vi "Teleop Intake Control.vi"(9 "D-Pad":T1, 10 "Button Cluster":T2, 11 "Axes":T3) -> ()   [LabVIEW 2017]
uses:
  Common Code/Gamepads/Axes Cluster.ctl
  Common Code/Gamepads/Button Cluster.ctl
  Common Code/Gamepads/D-Pad.ctl
  Common Code/Intake States.ctl
  Common Code/Intake Mode.ctl
  Common Code/Utilities/Change Detect.vi
  Robot Global Data.vi
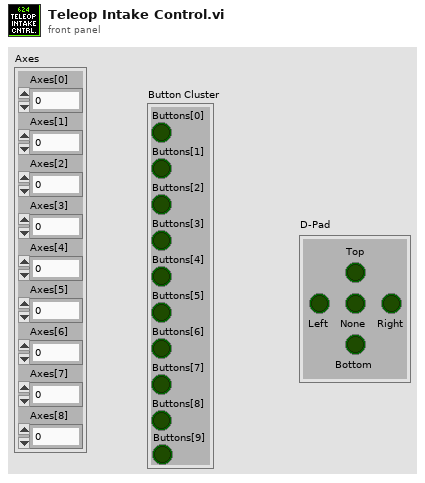
[diagram p1: front panel]
types:
  T1 = typedef "D-Pad.ctl" = cluster{"Top":bool, "Bottom":bool, "None":bool, "Right":bool, "Left":bool}
  T2 = typedef "Button Cluster.ctl" = cluster{"Buttons[0]":bool, "Buttons[1]":bool, "Buttons[2]":bool, "Buttons[3]":bool, "Buttons[4]":bool, "Buttons[5]":bool, "Buttons[6]":bool, "Buttons[7]":bool, "Buttons[8]":bool, "Buttons[9]":bool}
  T3 = typedef "Axes Cluster.ctl" = cluster{"Axes[0]":dbl, "Axes[1]":dbl, "Axes[2]":dbl, "Axes[3]":dbl, "Axes[4]":dbl, "Axes[5]":dbl, "Axes[6]":dbl, "Axes[7]":dbl, "Axes[8]":dbl}
  T4 = typedef "Intake States.ctl" = enum16{"Zero", "Override Angle", "Idle", "Drop Mid", "Drop Low", "Outtake", "Intake"}
  T5 = typedef "Intake Mode.ctl" = enum16{"Auto", "Semi Auto", "Manual"}
  T6 = typedef "Intake Command Cluster.ctl" = cluster{"Intake Mode":T5, "Intake States":T4, "Manual Roller Power":dbl, "Manual Close?":bool, "Manual Lift Power":dbl, "Override Lift?":bool, "Override Angle":dbl}
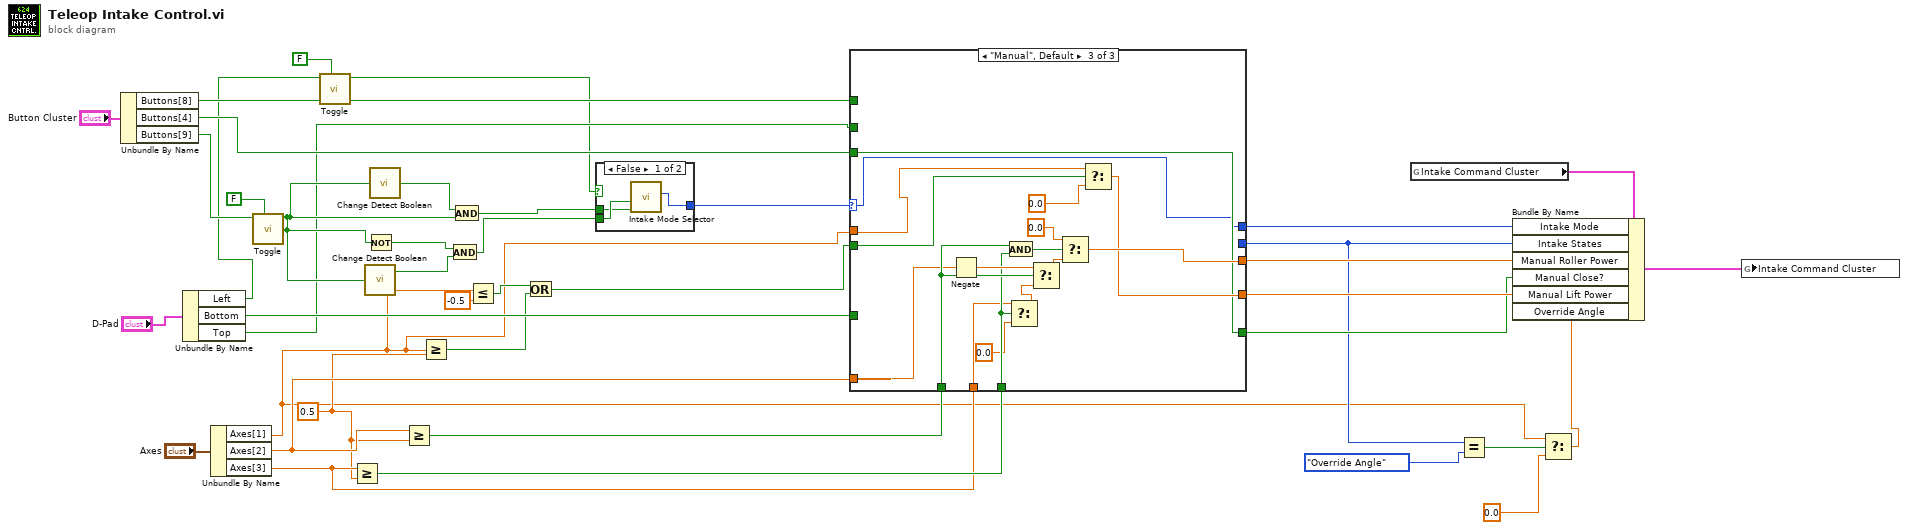
[diagram p0: block diagram]
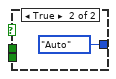
[diagram p2: hidden frame]
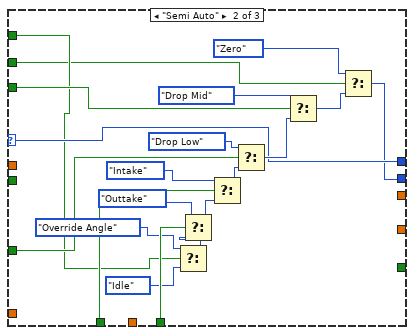
[diagram p4: hidden frame]
diagram:
  w22 = 0.5
  n1 = Unbundle By Name("Button Cluster") -> ("Buttons[8]"=w21:bool, "Buttons[4]"=w28:bool, "Buttons[9]"=w35:bool)
  n2 = Unbundle By Name("D-Pad") -> ("Left"=w1:bool, "Bottom"=w27:bool, "Top"=w7:bool)
  n3 = Unbundle By Name("Axes") -> ("Axes[1]"=w10:dbl, "Axes[2]"=w24:dbl, "Axes[3]"=w23:dbl)
  n4 = call "Toggle.vi"("Initial Value"=FALSE, "In"=w35) -> ("Toggled"=w30:bool)  [unwired: 9 in]
  n5 = call "Toggle.vi"("Initial Value"=FALSE, "In"=w1) -> ("Toggled"=w2:bool)  [unwired: 9 in]
  n6 = Greater Or Equal?(x=w23, y=w22) -> (x >= y?=w25:bool)
  n7 = call "Change Detect Boolean.vi"("In"=w30) -> ("Changed?"=w32:bool)
  n8 = Not(x=w30) -> (.not. x?=w31:bool)
  n9 = call "Change Detect Boolean.vi"("In"=w30) -> ("Changed?"=w33:bool)
  n10 = Greater Or Equal?(x=w24, y=w22) -> (x >= y?=w26:bool)
  n11 = Greater Or Equal?(x=w10, y=w22) -> (x >= y?=w19:bool)
  n12 = And(x=w31, y=w32) -> (x .and. y?=w6:bool)
  n13 = And(x=w33, y=w30) -> (x .and. y?=w5:bool)
  n14 = Less Or Equal?(x=w10, y=-0.5) -> (x <= y?=w18:bool)
  n15 = Or(x=w18, y=w19) -> (x .or. y?=w16:bool)
  n16 = case shown="False" w2 {
    tunnel: w6 -> [w43 _]
    tunnel: w5 -> [w42 _]
    tunnel: [w41 Intake_Mode."Auto" ("Intake Mode")] -> w4
    frame False {
      n17 = call "Intake Mode Selector.vi"("Semi Auto?"=w42, "Manual?"=w43) -> ("Intake Mode"=w41:T5)  [unwired: 9 in]
    }
    frame True {
    }
  }
  n18 = case shown="\"Manual\", Default" w4 {
    selector: w4 -> [w45 w52 w66]
    tunnel: [w45 w52 w66] -> w29
    tunnel: w28 -> [_ w64 w67]
    tunnel: w27 -> [_ w61 _]
    tunnel: w26 -> [_ w57 w80]
    tunnel: w25 -> [_ w55 w75]
    tunnel: w24 -> [_ _ w77]
    tunnel: w23 -> [_ _ w74]
    tunnel: [_ w51 _] -> w12
    tunnel: w16 -> [_ _ w71]
    tunnel: w10 -> [_ _ w70]
    tunnel: w21 -> [_ w50 _]
    tunnel: [_ _ w72] -> w20
    tunnel: [_ _ w68] -> w15
    tunnel: [_ _ w67] -> w14
    tunnel: w7 -> [_ w46 _]
    frame "Auto" {
    }
    frame "Semi Auto" {
      n19 = Select(t=Intake_States."Override Angle" ("Intake States"), s=w50, f=Intake_States."Idle" ("Intake States")) -> (s? t:f=w49:T4)
      n20 = Select(t=Intake_States."Outtake" ("Intake States"), s=w55, f=w49) -> (s? t:f=w54:T4)
      n21 = Select(t=Intake_States."Intake" ("Intake States"), s=w57, f=w54) -> (s? t:f=w53:T4)
      n22 = Select(t=Intake_States."Drop Low" ("Intake States"), s=w61, f=w53) -> (s? t:f=w60:T4)
      n23 = Select(t=Intake_States."Drop Mid" ("Intake States"), s=w64, f=w60) -> (s? t:f=w59:T4)
      n24 = Select(t=Intake_States."Zero" ("Intake States"), s=w46, f=w59) -> (s? t:f=w51:T4)
    }
    frame "Manual", Default {
      n25 = Negate(x=w77) -> (-x=w78:dbl)
      n26 = And(x=w80, y=w75) -> (x .and. y?=w81:bool)
      n27 = Select(t=w74, s=w75, f=0.0) -> (s? t:f=w76:dbl)
      n28 = Select(t=w78, s=w80, f=w76) -> (s? t:f=w79:dbl)
      n29 = Select(t=0.0, s=w81, f=w79) -> (s? t:f=w72:dbl)
      n30 = Select(t=w70, s=w71, f=0.0) -> (s? t:f=w68:dbl)
    }
  }
  n31 = global read "Robot Global Data.vi" "Intake Command Cluster"() -> (w39:T6)
  n32 = Equal?(x=w12, y=Intake_States."Override Angle" ("Intake States")) -> (x = y?=w13:bool)
  n33 = Select(t=w10, s=w13, f=0.0) -> (s? t:f=w8:dbl)
  n34 = Bundle By Name(cluster=w39, "Intake Mode"=w29, "Intake States"=w12, "Manual Roller Power"=w20, "Manual Close?"=w14, "Manual Lift Power"=w15, "Override Angle"=w8) -> (w38:T6)
  n35 = global write "Robot Global Data.vi" "Intake Command Cluster"(w38) -> ()
